vi "Pre Launch Init.vi"(11 "Nested in":refnum<class "Products Picker.lvclass">) -> (0 "error out":errorcluster, 3 "Nested out":refnum<class "Products Picker.lvclass">)   [LabVIEW 2020, in "Products Picker.lvlib" / "Products Picker.lvclass"]
doc: "(<B>Filename</B>: Actor Framework.lvlib:Actor.lvclass:Pre Launch Init.vi)\n\nDefines behavior that occurs after the Launch Nested Actor method is invoked but before the actor's Actor Core method begins running.\n\nBy default, this method does nothing. A descendant class may override it to define behavior."
uses:
  Products Picker.lvclass
  C:/Program Files (x86)/National Instruments/LabVIEW 2020/vi.lib/ActorFramework/Actor/Actor.lvclass
  Products Picker.lvclass/Products Picker.ctl
  <vilib>/ActorFramework/Actor/Actor.lvclass/Actor.ctl
  <vilib>/ActorFramework/Message Enqueuer/Message Enqueuer.lvclass/Message Enqueuer.ctl
  <vilib>/ActorFramework/Message Enqueuer/Init from Existing Queue.vi
  <vilib>/ActorFramework/Message Enqueuer/Enqueue.vi
  Products Picker Messages/Load Products Msg/Load Products Msg.lvclass
  C:/Program Files (x86)/National Instruments/LabVIEW 2020/vi.lib/ActorFramework/Message/Message.lvclass
  <vilib>/ActorFramework/Message Priority Queue/Priority Enqueue.vi
  <vilib>/ActorFramework/Message Enqueuer/Message Enqueuer.lvclass
  <vilib>/ActorFramework/Actor/Actor.lvclass
  Products Picker Messages/Update Display Msg/Update Display Msg.lvclass
  D:/Storage/Source Code/Clase AF/ClaseAF/05 AF Camera/Products Picker/Products Picker.lvclass
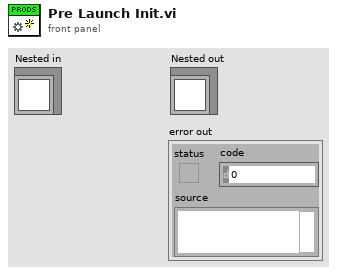
[diagram p1: front panel]
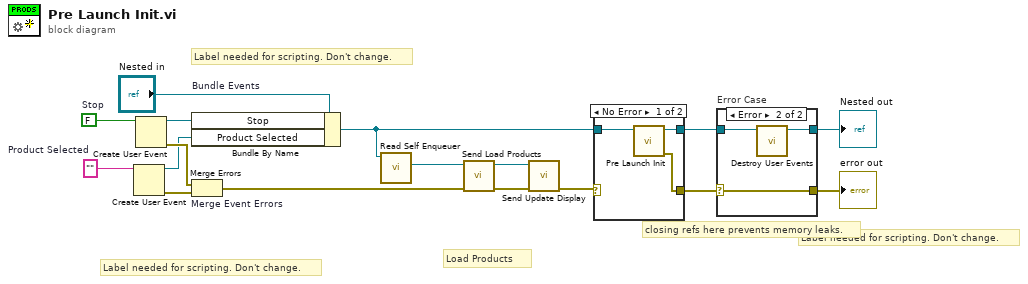
[diagram p0: block diagram]
diagram:
  w9 = ""  # Product Selected
  w16 = FALSE  # Stop
  # "Load Products"
  # "Label needed for scripting. Don't change."
  # "Label needed for scripting. Don't change."
  # "Label needed for scripting. Don't change."
  # "closing refs here prevents memory leaks."
  n1 = Create User Event(user event datatype=w9) -> (user event=w8:refnum<user-event>, error out=w7:errorcluster)  [unwired: 1 in]
  n2 = Create User Event(user event datatype=w16) -> (user event=w13:refnum<user-event>, error out=w15:errorcluster)  [unwired: 1 in]
  n3 = Bundle By Name "Bundle Events"(cluster="Nested in", "Stop"=w13, "Product Selected"=w8) -> (w6:refnum<class "Products Picker.lvclass">)
  n4 = Merge Errors "Merge Event Errors"(w15, w7) -> (w4:errorcluster)
  n5 = call <vilib>:"Read Self Enqueuer.vi"("Actor"=w6) -> ("Self Enqueuer"=w5:refnum<class "Message Enqueuer.lvclass">)  [unwired: 10 in]
  n6 = call "Send Load Products.vi"("error in (no error)"=w4, "Message Enqueuer"=w5) -> ("error out"=w3:errorcluster, "Message Enqueuer out"=w1:refnum<class "Message Enqueuer.lvclass">)  [unwired: 8 in]
  n7 = call "Send Update Display.vi"("error in (no error)"=w3, "Message Enqueuer"=w1) -> ("error out"=w2:errorcluster)  [unwired: 8 in, 1 out]
  n8 = case shown="No Error" w2 {
    selector: w2 -> [_ w22]
    tunnel: [w20 w21] -> w11
    tunnel: w6 -> [w19 w21]
    tunnel: [w18 w22] -> w10
    frame No Error {
      n9 = call-parent "Pre Launch Init.vi"("Actor in"=w19) -> ("error out"=w18:errorcluster, "Actor out"=w20:refnum<class "Products Picker.lvclass">)  [unwired: 9 in]
    }
    frame Error {
    }
  }
  n10 = case "Error Case" shown="Error" w10 {
    selector: w10 -> [w23 w27]
    tunnel: w11 -> [w24 w26]
    tunnel: [w24 w25] -> w14
    tunnel: [w23 w27] -> w12
    frame No Error {
    }
    frame Error {
      n11 = call "Destroy User Events.vi"("UI Template in"=w26) -> ("UI Template out"=w25:refnum<class "Products Picker.lvclass">)  [unwired: 10 in]
    }
  }
  "error out" <- w12
  "Nested out" <- w14
